vi "check syntax_core.vi"(8 "error in (no error)":errorcluster caption="에러 입력(에러 없음)", 11 "Script Line_i2c r 입력":refnum<class "Script Line_i2c r.lvclass">) -> (0 "error out":errorcluster caption="에러 출력", 3 "Script Line_i2c r 출력":refnum<class "Script Line_i2c r.lvclass">)   [LabVIEW 2020, in "Script Line_i2c r.lvclass"]
uses:
  Script Line_i2c r.lvclass
  Script Line/Script Line.lvclass/Script Line.ctl
  Script Line_i2c/Script Line_i2c.lvclass/Script Line_i2c.ctl
  Script Line_i2c/Accessors/Write slv.vi
  Script Line_i2c/Accessors/Write reg.vi
  Script Line/Accessors/Read parameter.vi
  Script Line/Accessors/Read parameter string index.vi
  Script Line/Script Line.lvclass
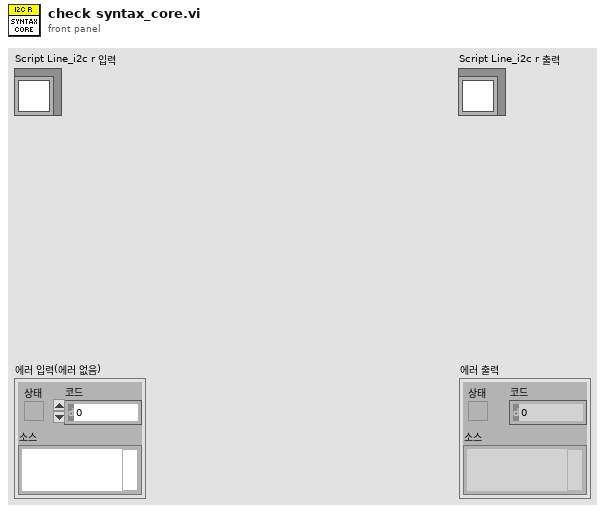
[diagram p1: front panel]
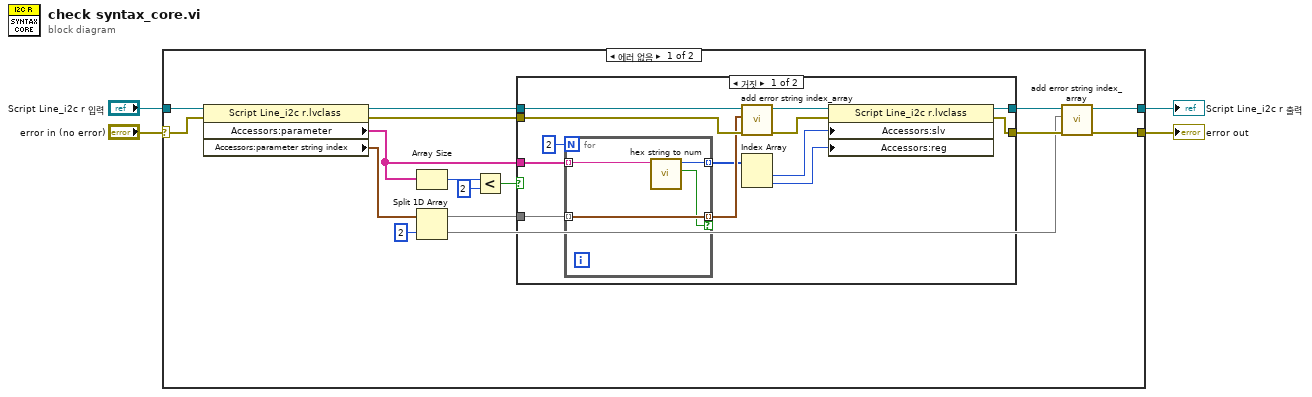
[diagram p0: block diagram]
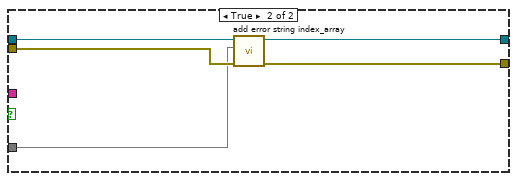
[diagram p2: hidden frame]
diagram:
  n1 = case shown="에러 없음" "error in (no error)" {
    selector: "error in (no error)" -> [w19 w44]
    tunnel: [w8 w44] -> w1
    tunnel: [w6 w43] -> w2
    tunnel: "Script Line_i2c r 입력" -> [w20 w43]
    frame No Error {
      n2 = property class="Script Line_i2c r.lvclass"(reference=w20, error in=w19) -> (reference out=w11:refnum<class "Script Line_i2c r.lvclass">, error out=w10:errorcluster, "Accessors:parameter"=w13:string[], "Accessors:parameter string index"=w15:cluster{"start":u32, "end":u32}[])
      n3 = Array Size(array=w13) -> (size(s)=w17:i32)
      n4 = Split 1D Array(array=w15, index=2 ("인덱스")) -> (first subarray=w12:cluster{"start":u32, "end":u32}[], second subarray=w5:cluster{"start":u32, "end":u32}[])
      n5 = Less?(x=w17, y=2) -> (x < y?=w14:bool)
      n6 = case shown="거짓" w14 {
        tunnel: w13 -> [w32 _]
        tunnel: w12 -> [w31 w38]
        tunnel: w11 -> [w33 w40]
        tunnel: w10 -> [w30 w42]
        tunnel: [w27 w41] -> w9
        tunnel: [w25 w39] -> w7
        frame False {
          n7 = for {
            N: 2 -> [_]
            tunnel: w32 -> [w37] mode=indexing
            tunnel: w31 -> [w35] mode=indexing
            tunnel: [w36] -> w24 mode=indexing
            tunnel: [w35] -> w28 mode=indexing if=w34
            n8 = call "hex string to num.vi"("string"=w37) -> ("error"=w34:bool, "num"=w36:u32)  [unwired: 7 in, 2 out]
          }
          n9 = call "add error string index_array.vi"("error in (no error)"=w30, "index_array"=w28, "Script Line 입력"=w33) -> ("error out"=w29:errorcluster, "Script Line 출력"=w26:refnum<class "Script Line_i2c r.lvclass">)  [unwired: 7 in]
          n10 = Index Array(array=w24) -> (element #1=w23:u32, element #2=w22:u32)  [unwired: 2 in]
          n11 = property class="Script Line_i2c r.lvclass"(reference=w26, error in=w29, "Accessors:slv"=w23, "Accessors:reg"=w22) -> (reference out=w25:refnum<class "Script Line_i2c r.lvclass">, error out=w27:errorcluster)
        }
        frame True {
          n12 = call "add error string index_array.vi"("error in (no error)"=w42, "index_array"=w38, "Script Line 입력"=w40) -> ("error out"=w41:errorcluster, "Script Line 출력"=w39:refnum<class "Script Line_i2c r.lvclass">)  [unwired: 7 in]
        }
      }
      n13 = call "add error string index_array.vi"("error in (no error)"=w9, "index_array"=w5, "Script Line 입력"=w7) -> ("error out"=w8:errorcluster, "Script Line 출력"=w6:refnum<class "Script Line_i2c r.lvclass">)  [unwired: 7 in]
    }
    frame Error {
    }
  }
  "error out" <- w1
  "Script Line_i2c r 출력" <- w2
